vi "ProducerConsumerEvents_Events_aula.vi"() -> ()   [LabVIEW 2026]
doc: "Use this template to build a producer/consumer design pattern with events to produce queue items. Use this design pattern instead of the User Interface Event Handler pattern for user interfaces when you want to execute code asynchronously in response to an event without slowing the user interface responsiveness."
uses:
  <vilib>/Instr/_visa.llb/VISA Configure Serial Port (Instr).vi
panel:
  in  "Enable Termination\nChar (T)":bool=TRUE
  in  "termination char\n(0xA = '\\n' = LF)":u8=10 format="%.0x"
  in  "flow control (0:none)":u16(ring) items=["None", "XON/XOFF", "RTS/CTS", "XON/XOFF & RTS/CTS", "DTR/DSR", "XON/XOFF & DTR/DSR"]
  in  "parity (0:none)":enum16{"None", "Odd", "Even", "Mark", "Space"}(ring)
  in  "data bits (8)":u16=8 min=5 max=8 step=1
  in  "baud rate (9600)":u32=9600
  in  "VISA resource name":refnum<visa-resource-name>
  in  "Read":bool
  in  "stop 3":bool
  in  "Write":bool
  in  "stop 2":bool
  out "Humidity":dbl(graph)
  out "Temperature":dbl(graph)
  in  "stop":bool
  out "read buffer":string
  out "error out":errorcluster
  in  "Read Count":u32=1000
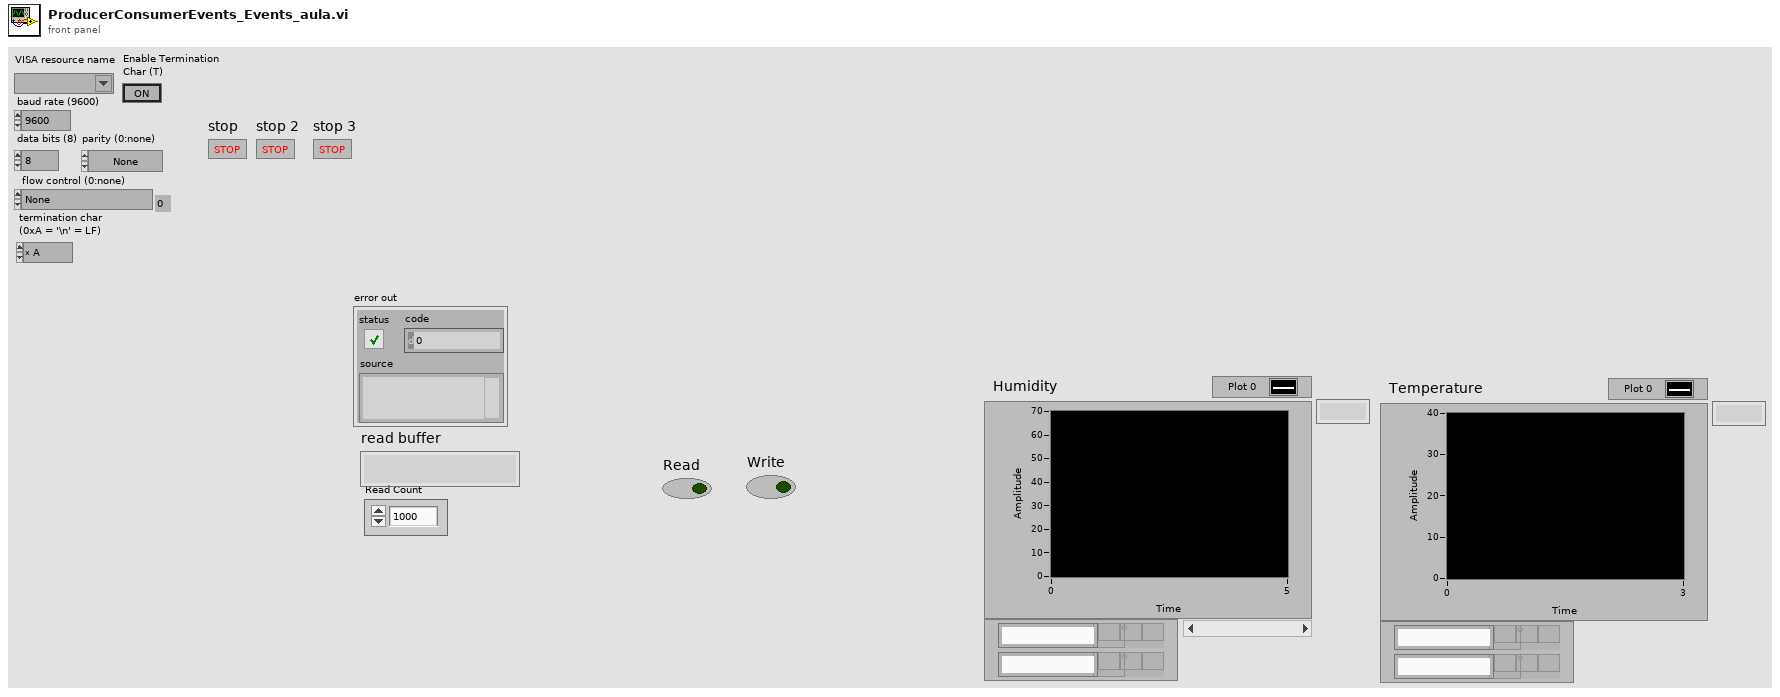
[diagram p1: front panel]
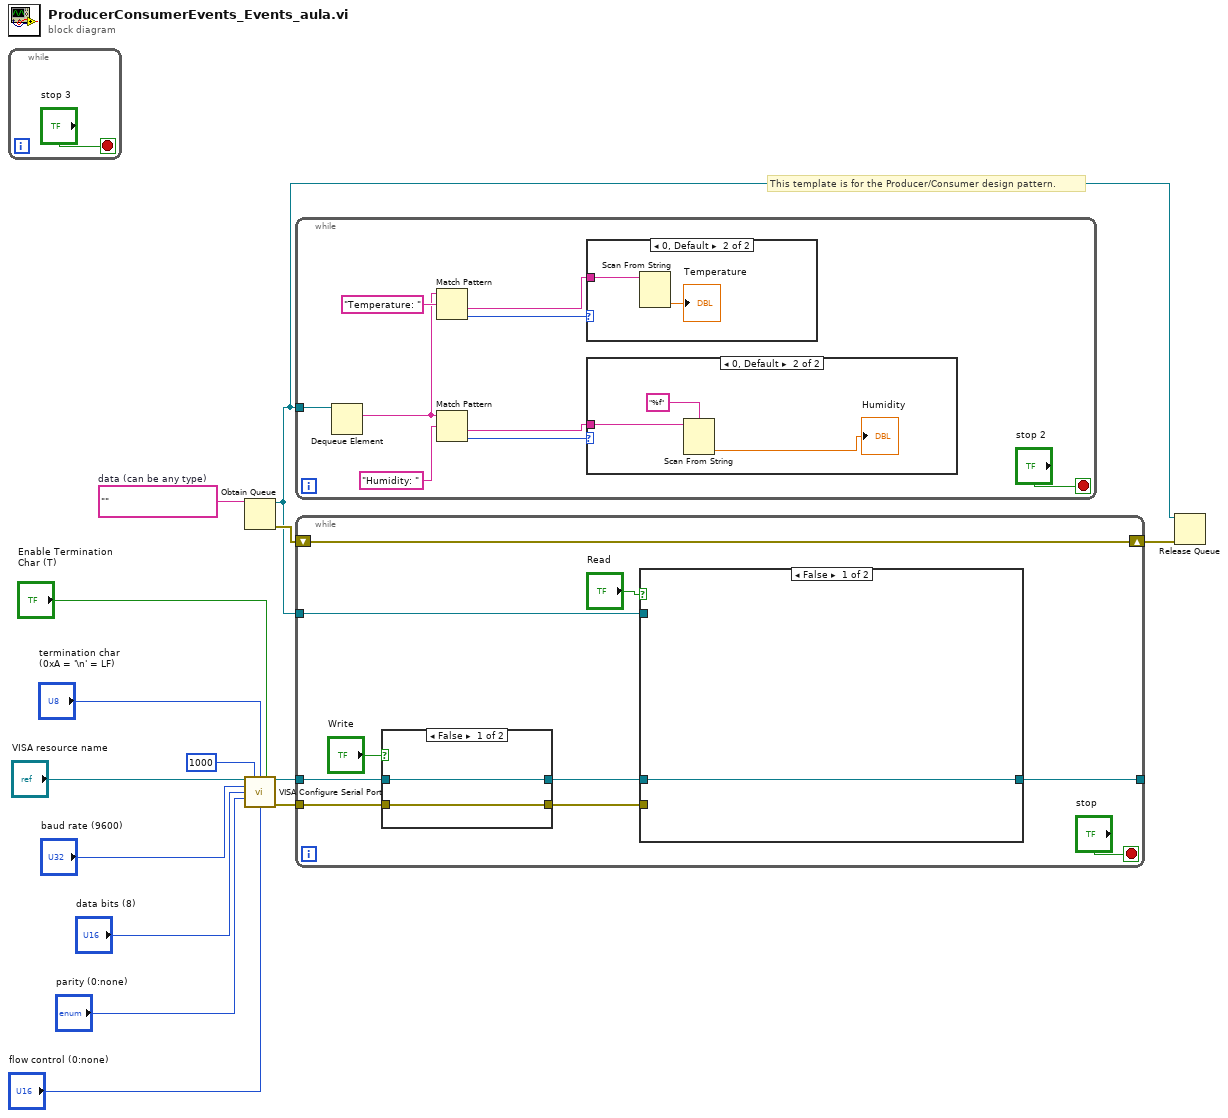
[diagram p0: block diagram]
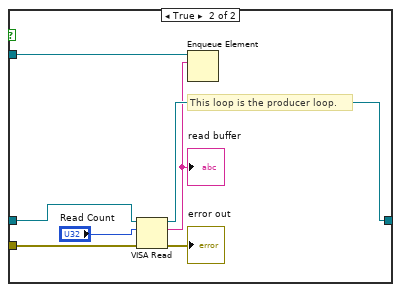
[diagram p4: hidden frame]
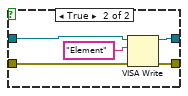
[diagram p5: hidden frame]
diagram:
  w9 = ""  # data (can be any type)
  # "This template is for the Producer/Consumer design pattern."
  n1 = while {
    stop <- "stop 3" stop-if-true
  }
  n2 = Obtain Queue(element data type=w9) -> (queue out=w12:refnum<queue>, error out=w14:errorcluster)  [unwired: 4 in, 1 out]
  n3 = call-poly "VISA Configure Serial Port"("VISA resource name"="VISA resource name", "timeout (10sec)"=u32 1000, "termination char\n(0xA = '\\n' = LF)"="termination char\n(0xA = '\\n' = LF)", "Enable Termination\nChar (T)"="Enable Termination\nChar (T)", "baud rate (9600)"="baud rate (9600)", "data bits (8)"="data bits (8)", "parity (0:none)"="parity (0:none)", "flow control (0:none)"="flow control (0:none)") -> ("VISA resource name out"=w11:refnum<visa-resource-name>, "error out"=w10:errorcluster)  [unwired: 2 in, 4 out]
  n4 = while {
    tunnel: w12 -> [w24]
    stop <- "stop 2" stop-if-true
    n5 = Dequeue Element(queue=w24) -> (element=w18:string)  [unwired: 2 in, 3 out]
    n6 = Match Pattern(string=w18, regular expression="Temperature: ") -> (after substring=w16:string, offset past match=w20:i32)  [unwired: 1 in, 2 out]
    n7 = Match Pattern(string=w18, regular expression="Humidity: ") -> (after substring=w21:string, offset past match=w19:i32)  [unwired: 1 in, 2 out]
    n8 = case shown="0, Default" w20 {
      tunnel: w16 -> [_ w28]
      frame -1 {
      }
      frame 0, Default {
        n9 = Scan From String(input string=w28) -> (output 1=→"Temperature":dbl)  [unwired: 4 in, 3 out]
      }
    }
    n10 = case shown="0, Default" w19 {
      tunnel: w21 -> [_ w26]
      frame -1 {
      }
      frame 0, Default {
        n11 = Scan From String "Scan From String"(format string="%f", input string=w26) -> (output 1=→"Humidity":dbl)  [unwired: 3 in, 3 out]
      }
    }
  }
  n12 = while {
    shift-right: [w36] -> w13
    shift-left: w14 -> [w36]
    tunnel: w12 -> [w38]
    tunnel: [w39] -> _
    tunnel: w11 -> [w35]
    tunnel: w10 -> [w34]
    stop <- "stop" stop-if-true
    n13 = case shown="False" "Write" {
      tunnel: w35 -> [w49 w54]
      tunnel: w34 -> [w48 w53]
      tunnel: [w49 w52] -> w31
      tunnel: [w48 w51] -> w33
      frame False {
      }
      frame True {
        n14 = VISA Write(VISA resource name=w54, write buffer="Element", error in (no error)=w53) -> (VISA resource name out=w52:refnum<visa-resource-name>, error out=w51:errorcluster)  [unwired: 1 out]
      }
    }
    n15 = case shown="False" "Read" {
      tunnel: [w40 w46] -> w39
      tunnel: w38 -> [_ w43]
      tunnel: w33 -> [_ w42]
      tunnel: w31 -> [w40 w41]
      frame False {
      }
      frame True {
        # "This loop is the producer loop."
        n16 = VISA Read(VISA resource name=w41, byte count="Read Count", error in (no error)=w42) -> (VISA resource name out=w46:refnum<visa-resource-name>, read buffer=w44:string, error out=→"error out":errorcluster)  [unwired: 1 out]
        "read buffer" <- w44
        n17 = Enqueue Element(queue=w43, element=w44) -> ()  [unwired: 2 in, 3 out]
      }
    }
  }
  n18 = Release Queue(queue=w12, error in (no error)=w13) -> ()  [unwired: 1 in, 3 out]
